vi "GetRequestInfoForLog.vi"(1 "Log":T1) -> (0 "String":string)   [LabVIEW 2015]
doc: "Gets info for request topic or node"
uses:
  Console/Servers/ServerSubs/ROSLog.ctl
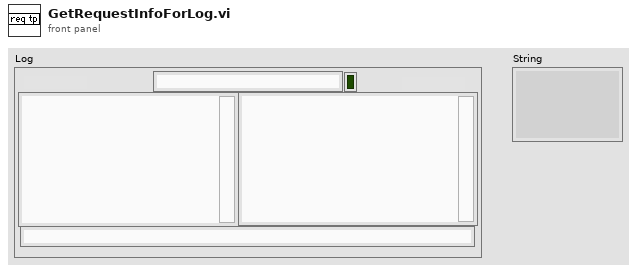
[diagram p1: front panel]
types:
  T1 = typedef "ROSLog.ctl" = cluster{"Sent":string, "Reply":string, "MethodName":string, "success":bool, "Dir1":string, "Dir2":string, "Time Stamp":string, "error":errorcluster, "Preamble":string, "Midamble":string, "Postamble":string}
  T2 = cluster{"Caller ID":string, "Topic Name":string, "Protocol":string, "URI":string, "ID":refnum<k5>}
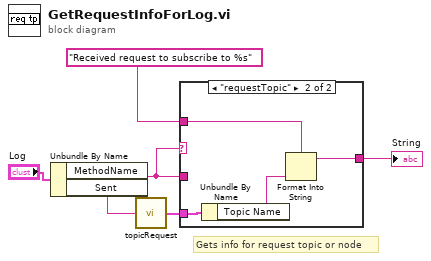
[diagram p0: block diagram]
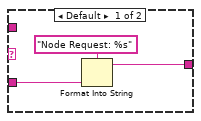
[diagram p2: hidden frame]
diagram:
  # "Gets info for request topic or node"
  n1 = Unbundle By Name("Log") -> ("MethodName"=w4:string, "Sent"=w3:string)
  n2 = call "topicRequest.vi"("XML"=w3) -> ("Subscriber"=w2:T2)
  n3 = case shown="\"requestTopic\"" w4 {
    tunnel: [w9 w13] -> w6
    tunnel: w4 -> [w8 _]
    tunnel: w2 -> [_ w12]
    tunnel: "Received request to subscribe to %s" ("format string") -> [_ w10]
    frame Default {
      n4 = Format Into String(format string="Node Request: %s", w8) -> (resulting string=w9:string)  [unwired: 2 in, 1 out]
    }
    frame "requestTopic" {
      n5 = Unbundle By Name(w12) -> ("Topic Name"=w11:string)
      n6 = Format Into String(format string=w10, w11) -> (resulting string=w13:string)  [unwired: 2 in, 1 out]
    }
  }
  "String" <- w6
